vi "LY.vi"() -> ()   [LabVIEW 2020]
panel:
  in  "LY":dbl
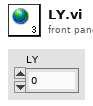
[diagram p1: front panel]
diagram:
